vi "Write Abort.vi"(8 "error in (no error)":errorcluster, 10 "Abort":bool, 11 "Process State Data in":refnum<class "Process State Data.lvclass">) -> (0 "error out":errorcluster, 3 "Process State Data out":refnum<class "Process State Data.lvclass">)   [LabVIEW 2022 SP3, in "Process State Data.lvclass"]
uses:
  Process State Data.lvclass
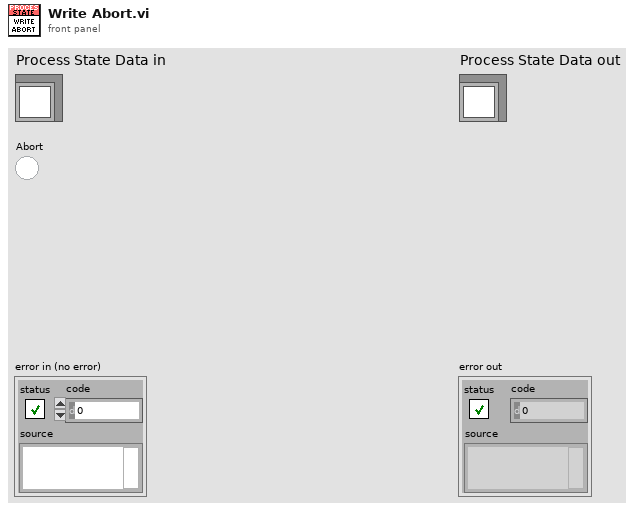
[diagram p1: front panel]
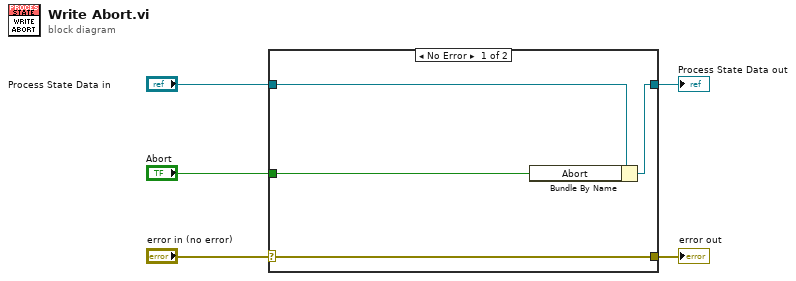
[diagram p0: block diagram]
diagram:
  n1 = case shown="No Error" "error in (no error)" {
    selector: "error in (no error)" -> [w9 w10]
    tunnel: [w9 w10] -> w4
    tunnel: [w7 w11] -> w2
    tunnel: "Process State Data in" -> [w8 w11]
    tunnel: "Abort" -> [w6 _]
    frame No Error {
      n2 = Bundle By Name(cluster=w8, "Abort"=w6) -> (w7:refnum<class "Process State Data.lvclass">)
    }
    frame Error {
    }
  }
  "error out" <- w4
  "Process State Data out" <- w2
